vi "Search from PRN  & Replacement Data1.vi"(0 "PRN  Call File":string="﻿\u0010CT~~CD,~CC^~CT~\n^XA~TA000~JSN^LT0^MNW^MTT^PON^PMN^LH0,0^JMA^PR3,3~SD22^JUS^LRN^CI0^XZ\n^XA\n^MMT\n^PW1200\n^LL0300\n^LS0\n^FT44,48^AAN,54,20^FH\\^FDAUTHENTIC ENGINEERS^FS\n^BY4,3,139^FT61,196^BCN,,Y,N\n^FD>;050620151983^FS\n^PQ1,0,1,Y^XZ\n", 2 "Model":string, 3 "Serial no":string) -> (7 "PRN out":string, 8 "Barcode Serial No":string="290915")   [LabVIEW 2015]
panel:
  out "result string 4":string
  out "result string 2":string
  out "substring":string
  # "﻿CT~~CD,~CC^~CT~\n^XA~TA000~JSN^LT0^MNW^MTD^PON^PMN^LH0,0^JMA^PR4,4~SD15^JUS^LRN^CI0^XZ\n^XA\n^MMT\n^PW320\n^LL0120\n^LS0\n^FT29,79^A0N,17,16^FH\\^FDMFR:1234^FS\n^FT30,56^A0N,17,16^FH\\^FDLNR:12234^FS\n^FT30,34^A0N,17,16^FH\\^FDajay kumar^FS\n^FT241,123^BQN,2,3\n^FH\\^FDMA,ajay kumarMFR:1234 LNR:12234^FS\n^PQ1,0,1,Y^XZ"
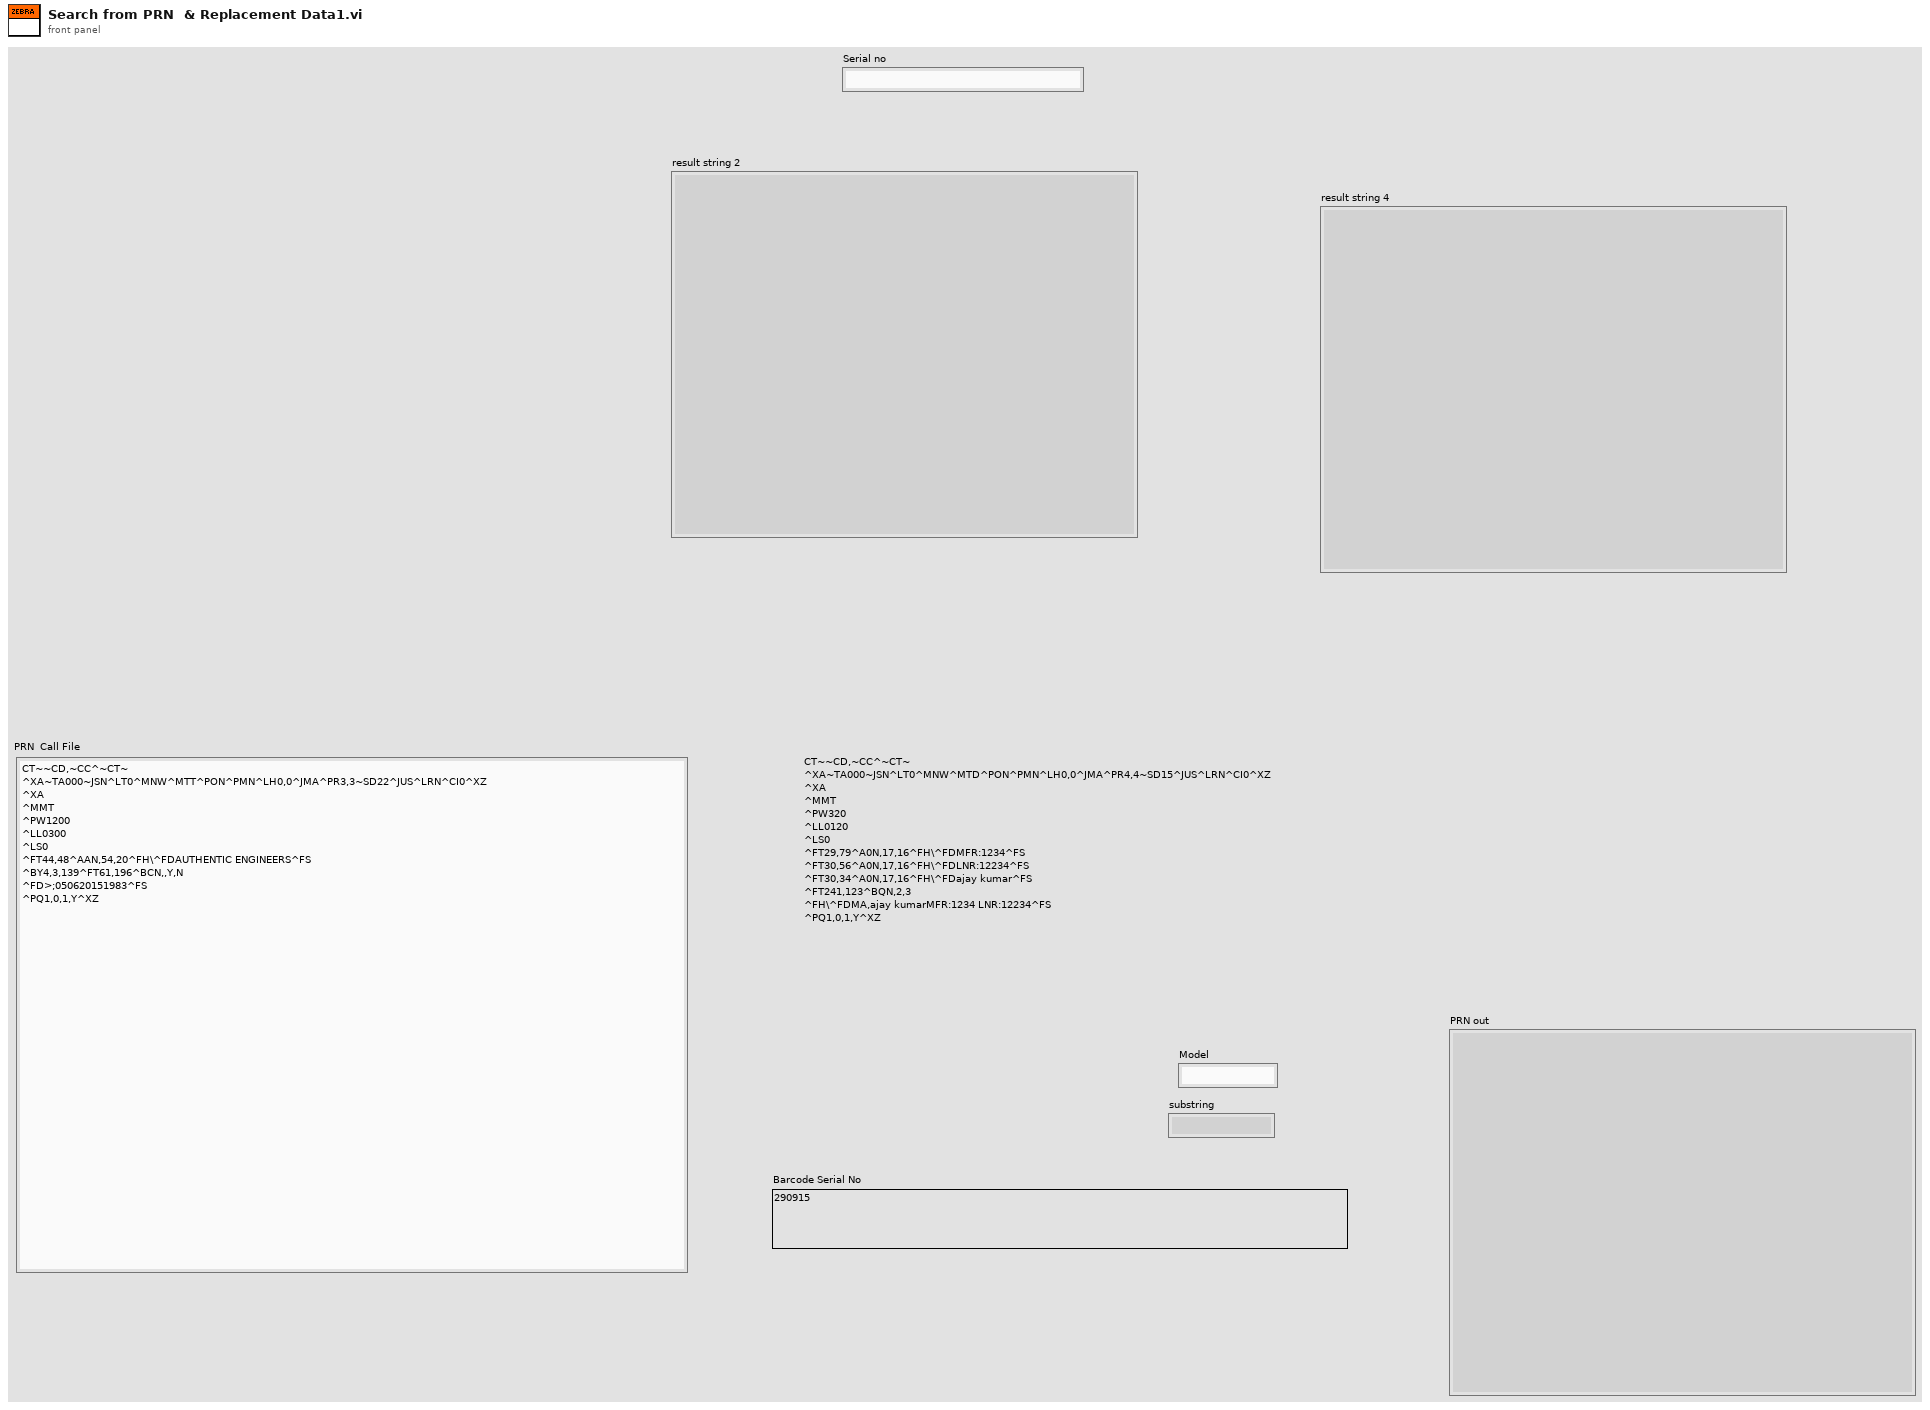
[diagram p1: front panel]
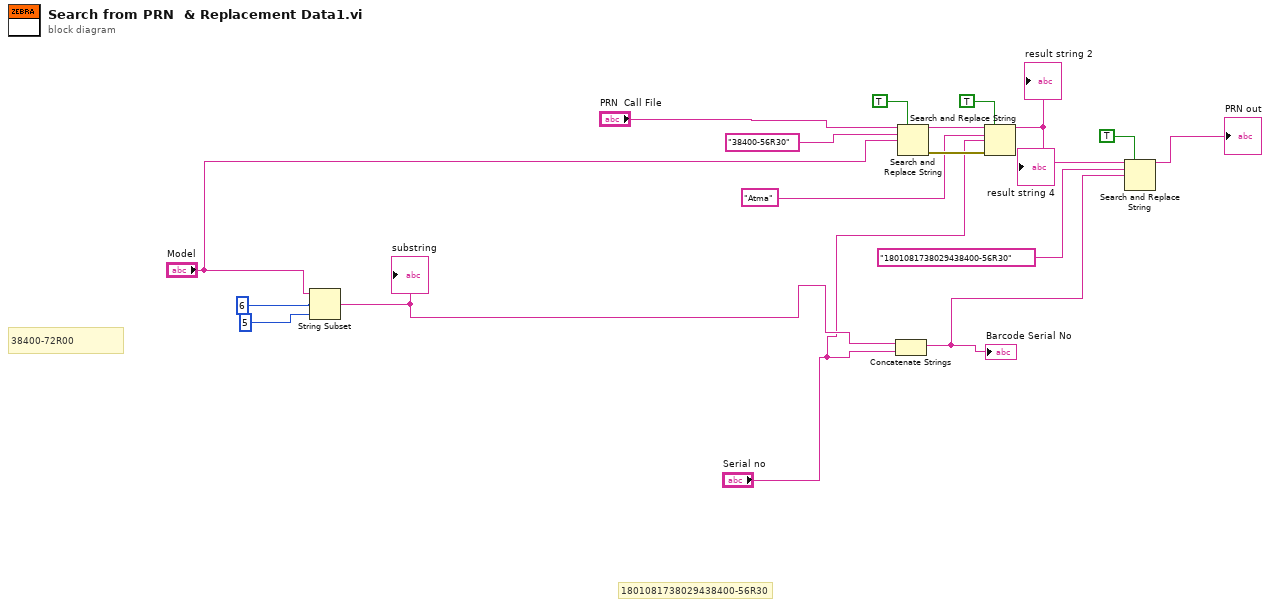
[diagram p0: block diagram]
diagram:
  # "1801081738029438400-56R30"
  # "38400-72R00"
  n1 = String Subset(string="Model", offset (0)=6, length (rest)=5 ("length (rest)")) -> (substring=w10:string)
  "substring" <- w10
  n2 = Concatenate Strings(w10, "Serial no") -> (w2:string)
  "Barcode Serial No" <- w2
  n3 = Search and Replace String(replace all?=TRUE ("replace all? (F)"), input string="PRN  Call File", search string="38400-56R30", replace string="Model") -> (result string=w16:string, error out=w15:errorcluster)  [unwired: 4 in, 2 out]
  n4 = Search and Replace String(replace all?=TRUE ("replace all? (F)"), input string=w16, search string="Atma" ("regular expression (\"\")"), replace string="Serial no", error in=w15) -> (result string=w5:string)  [unwired: 3 in, 3 out]
  "result string 2" <- w5
  n5 = Search and Replace String(replace all?=TRUE ("replace all? (F)"), input string=w5, search string="1801081738029438400-56R30" ("regular expression (\"\")"), replace string=w2) -> (result string=→"PRN out":string)  [unwired: 4 in, 3 out]
